vi "Configure PID Set.vi"(0 "VISA resource name":refnum<visa-resource-name>, 1 "Set (1)":i16=1, 2 "Channels (0: A)":i16(ring) items=["A", "B"], 3 "Proportional Band (25.0)":dbl=25.0 format="%.2f", 4 "Integral/Reset (0.0)":dbl format="%.2f", 5 "error in (no error)":errorcluster {"code" format="%.0x"}, 6 "Unit Address (1)":i16=1, 8 "Derivative/Rate (0.0)":dbl format="%.2f", 10 "Dead Band (0.0)":dbl format="%.2f", 12 "Hysteresis (3.0)":dbl=3.0 format="%.2f") -> (14 "VISA resource name out":refnum<visa-resource-name>, 19 "error out":errorcluster {"code" format="%.0x"})   [LabVIEW 2010]
doc: "This VI configures PID sets."
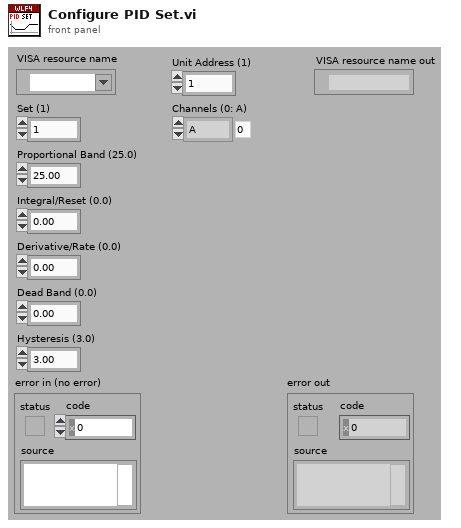
[diagram p1: front panel]
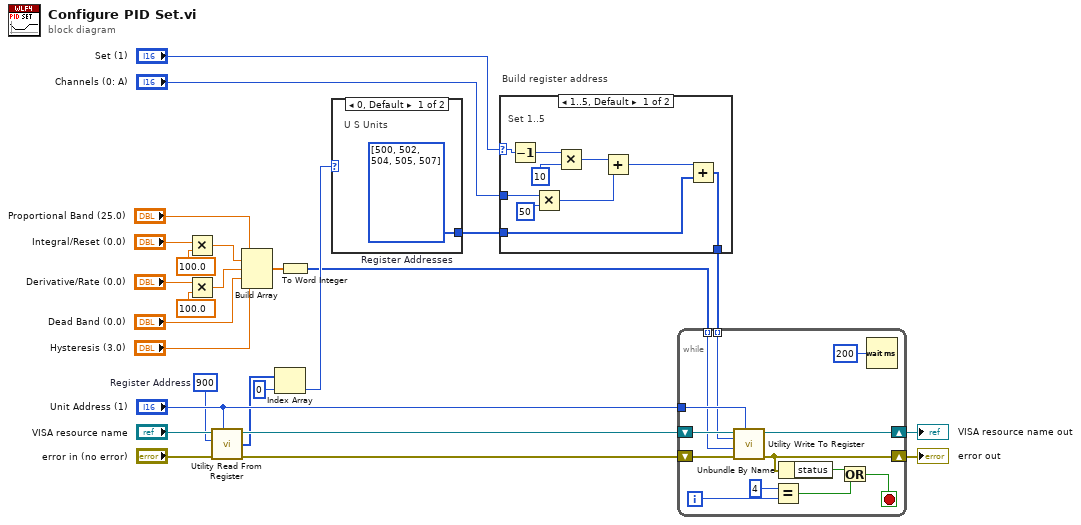
[diagram p0: block diagram]
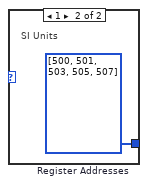
[diagram p2: hidden frame]
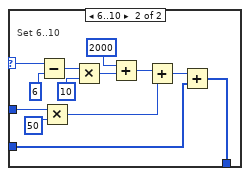
[diagram p3: hidden frame]
diagram:
  w16 = u16 900  # Register Address
  # "Build register address"
  n1 = Multiply(x="Integral/Reset (0.0)", y=100.0) -> (x*y=w3:dbl)
  n2 = Multiply(x="Derivative/Rate (0.0)", y=100.0) -> (x*y=w8:dbl)
  n3 = call "Utility Read From Register.vi"("Unit Address (1)"="Unit Address (1)", "error in (no error)"="error in (no error)", "Register Address (0)"=w16, "VISA resource name"="VISA resource name") -> ("error out"=w20:errorcluster, "Data"=w14:i16[], "VISA resource name out"=w19:refnum<visa-resource-name>)  [unwired: 5 in]
  n4 = Build Array("Proportional Band (25.0)", w3, w8, "Dead Band (0.0)", "Hysteresis (3.0)") -> (w5:dbl[])
  n5 = Index Array(array=w14, index=0) -> (element=w13:i16)
  n6 = To Word Integer(number=w5) -> (16bit integer=w1:i16[])
  n7 = case shown="0, Default" w13 {
    tunnel: [w27 w28] -> w12
    frame 0, Default {
      w27 = i32[] [500, 502, 504, 505, 507]  # Register Addresses
      # "U S Units"
    }
    frame 1 {
      w28 = i32[] [500, 501, 503, 505, 507]  # Register Addresses
      # "SI Units"
    }
  }
  n8 = case shown="1..5, Default" "Set (1)" {
    selector: "Set (1)" -> [w35 w46]
    tunnel: [w38 w51] -> w23
    tunnel: w12 -> [w34 w45]
    tunnel: "Channels (0: A)" -> [w32 w42]
    frame 1..5, Default {
      # "Set 1..5"
      n9 = Decrement(x=w35) -> (x-1=w36:i16)
      n10 = Multiply(x=w32, y=i16 50) -> (x*y=w30:i16)
      n11 = Multiply(x=w36, y=i16 10) -> (x*y=w31:i16)
      n12 = Add(x=w31, y=w30) -> (x+y=w29:i16)
      n13 = Add(x=w29, y=w34) -> (x+y=w38:i32[])
    }
    frame 6..10 {
      # "Set 6..10"
      n14 = Subtract(x=w46, y=i16 6) -> (x-y=w49:i16)
      n15 = Multiply(x=w42, y=i16 50) -> (x*y=w39:i16)
      n16 = Multiply(x=w49, y=i16 10) -> (x*y=w48:i16)
      n17 = Add(x=i16 2000, y=w48) -> (x+y=w40:i16)
      n18 = Add(x=w40, y=w39) -> (x+y=w44:i16)
      n19 = Add(x=w44, y=w45) -> (x+y=w51:i32[])
    }
  }
  n20 = while {
    tunnel: "Unit Address (1)" -> [w64]
    shift-right: [w61] -> w26
    shift-left: w19 -> [w63]
    shift-right: [w58] -> w25
    shift-left: w20 -> [w62]
    tunnel: w23 -> [w59] mode=indexing
    tunnel: w1 -> [w52] mode=indexing
    i -> [w55]
    stop <- w56 stop-if-true
    n21 = call "Utility Write To Register.vi"("Unit Address (1)"=w64, "error in (no error)"=w62, "Data (0)"=w52, "Register Address (0)"=w59, "VISA resource name"=w63) -> ("error out"=w58:errorcluster, "VISA resource name out"=w61:refnum<visa-resource-name>)  [unwired: 5 in]
    n22 = Equal?(x=4, y=w55) -> (x = y?=w53:bool)
    n23 = Unbundle By Name(w58) -> ("status"=w57:bool)
    n24 = Or(x=w57, y=w53) -> (x .or. y?=w56:bool)
    n25 = Wait (ms)(milliseconds to wait=u32 200) -> ()  [unwired: 1 out]
  }
  "error out" <- w25
  "VISA resource name out" <- w26
